vi "Insight_Laser_Close.vi"(8 "error in (no error)":errorcluster, 10 "VISA resource name":refnum<visa-resource-name>, 11 "connection ID":refnum<k5>) -> (0 "error out":errorcluster)   [LabVIEW 2010]
doc: "Insight Photonic Solutions\n\nThis VI closes the connection to the Insight Laser. The VI closes either Serial or TCP/IP connections.\n\nver 1.0 - original release"
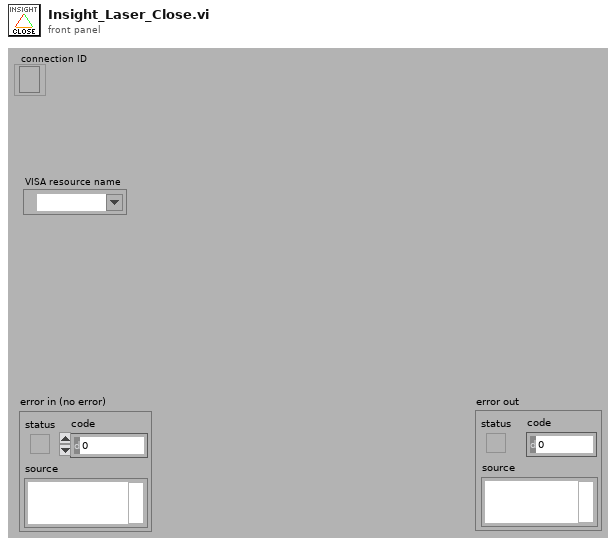
[diagram p1: front panel]
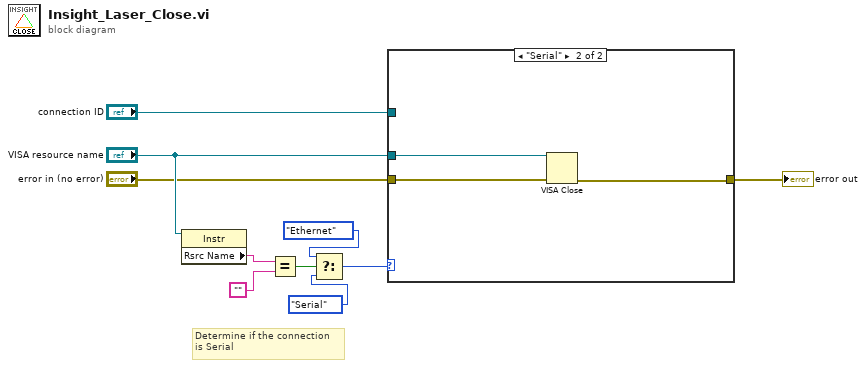
[diagram p0: block diagram]
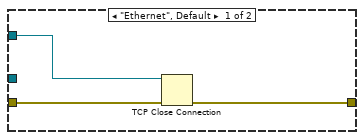
[diagram p2: hidden frame]
diagram:
  # "Determine if the connection\nis Serial"
  n1 = property class="Instr"(reference="VISA resource name") -> ("Rsrc Name"=w10:string)  [unwired: 1 in, 2 out]
  n2 = Equal?(x=w10, y="") -> (x = y?=w8:bool)
  n3 = Select(t=enum16{"Ethernet", "Serial"}."Ethernet", s=w8, f=enum16{"Ethernet", "Serial"}."Serial") -> (s? t:f=w5:enum16{"Ethernet", "Serial"})
  n4 = case shown="\"Serial\"" w5 {
    tunnel: [w12 w14] -> w3
    tunnel: "VISA resource name" -> [_ w15]
    tunnel: "error in (no error)" -> [w13 w16]
    tunnel: "connection ID" -> [w11 _]
    frame "Ethernet", Default {
      n5 = TCP Close Connection(connection ID=w11, error in (no error)=w13) -> (error out=w12:errorcluster)  [unwired: 1 in, 1 out]
    }
    frame "Serial" {
      n6 = VISA Close(VISA resource name=w15, error in (no error)=w16) -> (error out=w14:errorcluster)
    }
  }
  "error out" <- w3
